vi "New Version Num.vi"(8 "error in":errorcluster, 11 "build modified":T1={"App Name"="", "Build Type"=enum."Fix", "Current Version"="", "Next Version"="", "Check"=FALSE}) -> (0 "error IO":errorcluster, 3 "build modified out":T1={"App Name"="", "Build Type"=enum."Fix", "Current Version"="", "Next Version"="", "Check"=FALSE})   [LabVIEW 2025, in "App-Builder Library.lvlib" / "GUI Builder.lvclass"]
uses:
  GUI Builder.lvclass
  Builder/App descriptions.ctl
  Builder/Build Type.ctl
  Builder/Builder.lvclass
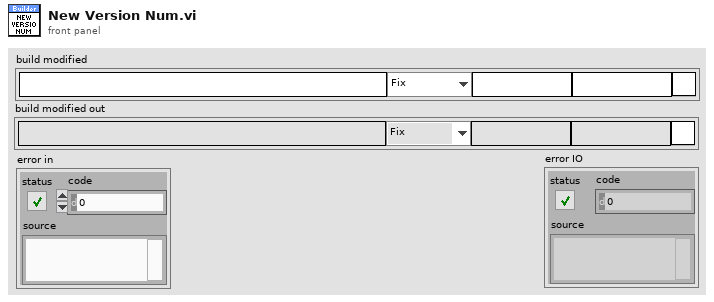
[diagram p1: front panel]
types:
  T1 = typedef "App-Builder Library.lvlib/Builder.lvclass/App descriptions.ctl" = cluster{"App Name":string, "Build Type":T2, "Current Version":string, "Next Version":string, "Check":bool}
  T2 = typedef "App-Builder Library.lvlib/Builder.lvclass/Build Type.ctl" = enum16{"Major", "Minor", "Fix", "Build"}
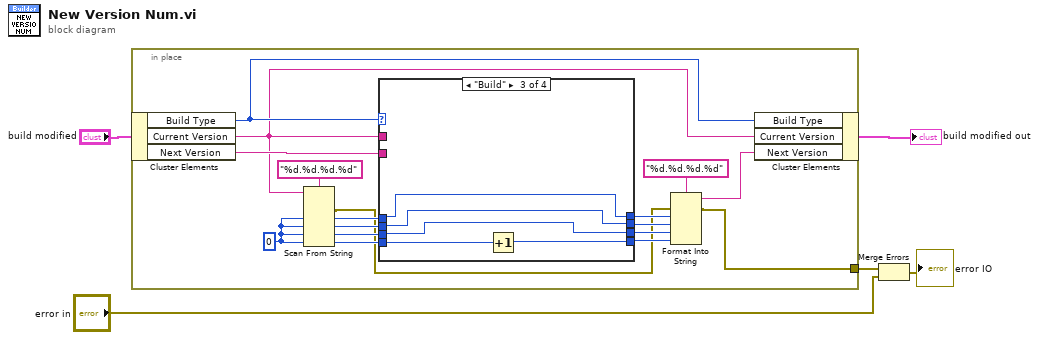
[diagram p0: block diagram]
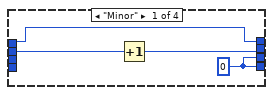
[diagram p2: hidden frame]
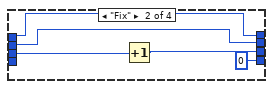
[diagram p3: hidden frame]
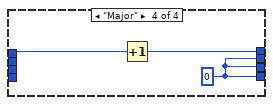
[diagram p4: hidden frame]
diagram:
  n1 = in-place {
    in-place-border: [w6] -> w3
    w13 = u16 0 ("x+1")
    n2 = in-place-cluster #1("build modified") -> ("Build Type"=w21:T2, "Current Version"=w19:string, "Next Version"=w22:string)
    n3 = Scan From String(format string="%d.%d.%d.%d", input string=w19, default 1=w13, default 2=w13, default 3=w13, default 4=w13) -> (error out=w7:errorcluster, output 1=w18:u16, output 2=w17:u16, output 3=w16:u16, output 4=w15:u16)  [unwired: 2 in, 2 out]
    n4 = case shown="\"Build\"" w21 {
      tunnel: w19 -> [_ _ _ _]
      tunnel: w22 -> [_ _ _ _]
      tunnel: w18 -> [w26 w29 w36 w39]
      tunnel: w17 -> [w24 w28 w35 _]
      tunnel: w16 -> [_ w31 w32 _]
      tunnel: w15 -> [_ _ w34 _]
      tunnel: [w26 w29 w36 w38] -> w11
      tunnel: [w25 u16 0 ("x+1") w33 w37] -> w10
      tunnel: [w25 w30 w32 w37] -> w9
      tunnel: [w23 w28 w35 w37] -> w8
      frame "Minor" {
        w25 = u16 0 ("x+1")
        n5 = Increment(x=w24) -> (x+1=w23:u16)
      }
      frame "Fix" {
        n6 = Increment(x=w31) -> (x+1=w30:u16)
      }
      frame "Build" {
        n7 = Increment(x=w34) -> (x+1=w33:u16)
      }
      frame "Major" {
        w37 = u16 0 ("x+1")
        n8 = Increment(x=w39) -> (x+1=w38:u16)
      }
    }
    n9 = Format Into String(format string="%d.%d.%d.%d", error in=w7, w11, w8, w9, w10) -> (resulting string=w12:string, error out=w6:errorcluster)  [unwired: 1 in]
    n10 = in-place-cluster #1("Build Type"=w21, "Current Version"=w19, "Next Version"=w12) -> (→"build modified out":T1)
  }
  n11 = Merge Errors(w3, "error in") -> (→"error IO":errorcluster)
